vi "Autonomous_Load.vi"(0 "Number of Commands":i32, 5 "Subsystems":string[](array[string]), 7 "Commands":string[](array[string]), 9 "Inputs":string[][](array[string]), 11 "error in":errorcluster) -> (4 "Queue_Key":refnum<queue>, 6 "Autonomous_Queue":refnum<queue>, 15 "errror out":errorcluster)   [LabVIEW 2019]
uses:
  Queue_Key_Data.ctl
  Robot_Subsystems.ctl
  Subsystems/Drive/Drive_Cluster.ctl
  Subsystems/Drive/Drive_Control_States.ctl
  Subsystems/Drive/Drive_Orientation_States.ctl
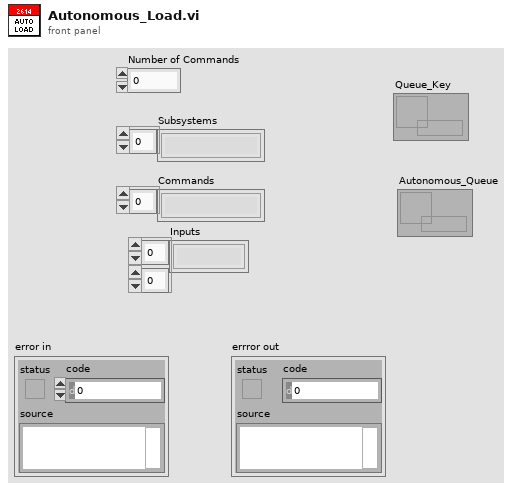
[diagram p1: front panel]
types:
  T1 = typedef "Robot_Subsystems.ctl" = cluster{"Drive_Cluster":T2}
  T2 = typedef "Drive_Cluster.ctl" = cluster{"Control_State":T3, "Vertical_Throttle":dbl, "Lateral_Throttle":dbl, "Rotational_Throttle":dbl, "Strafe_In_Deadband":bool, "Rotation_In_Deadband":bool, "Orientation_State":T4, "Parameters":dbl[], "Step":i32, "Auto_Notifier":refnum<notifier>}
  T3 = typedef "Drive_Control_States.ctl" = enum16{"Manual_Control", "Command_DriveDistanceAtAngle", ""}
  T4 = typedef "Drive_Orientation_States.ctl" = enum16{"Robot-Oriented", "Field-Oriented"}
  T5 = typedef "Queue_Key_Data.ctl" = cluster{"Operation Notifier":refnum<notifier>, "Subsystem":string, "Concurrent":bool}
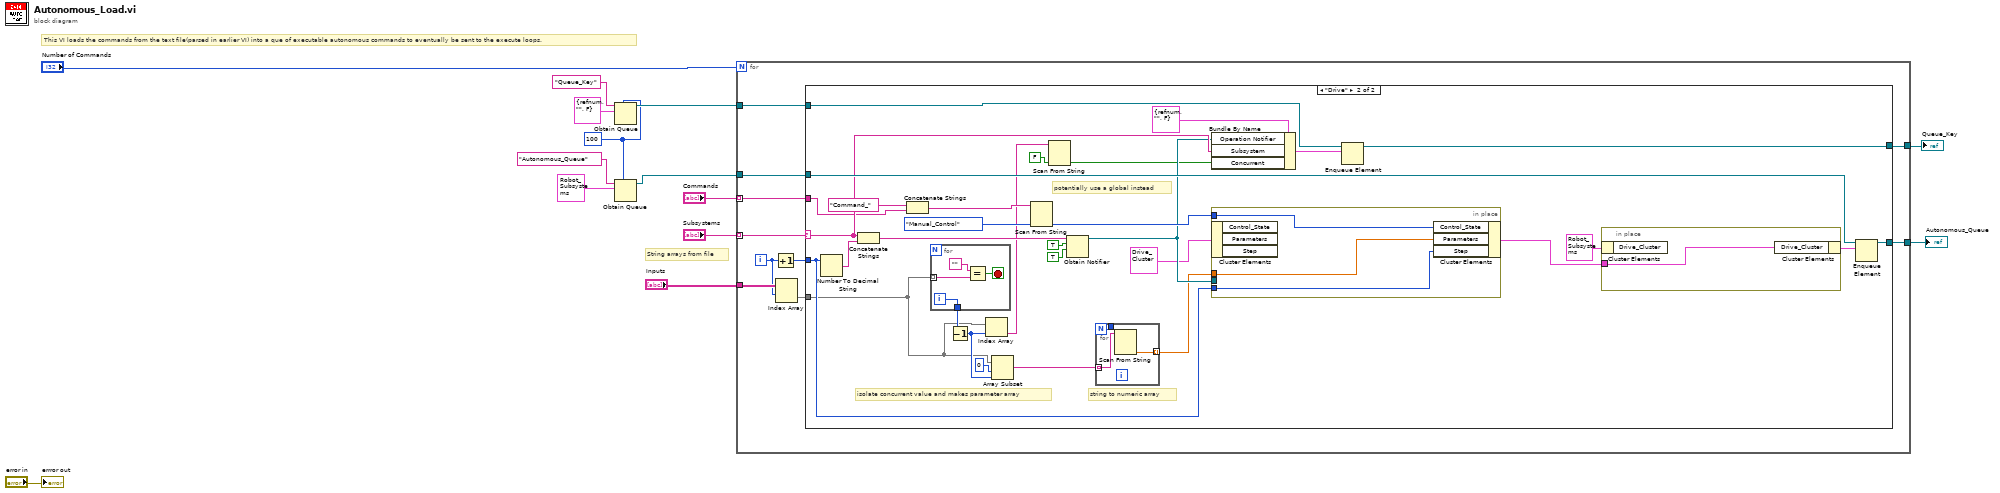
[diagram p0: block diagram]
diagram:
  w6 = 100 ("max queue size (-1, unlimited)")
  # "This VI loads the commands from the text file(parsed in earlier VI) into a que of executable autonomous commands to eventually be sent to the execute loops."
  # "String arrays from file"
  n1 = Obtain Queue(max queue size (-1, unlimited)=w6, name (unnamed)="Queue_Key", element data type=T5 {"Operation Notifier"=refnum, "Subsystem"="", "Concurrent"=FALSE} ("Queue Key Data")) -> (queue out=w12:refnum<queue>)  [unwired: 2 in, 2 out]
  n2 = Obtain Queue(max queue size (-1, unlimited)=w6, name (unnamed)="Autonomous_Queue", element data type=T1 {"Drive_Cluster"={"Control_State"=enum."Manual_Control", "Vertical_Throttle"=0.0, "Lateral_Throttle"=0.0, "Rotational_Throttle"=0.0, "Strafe_In_Deadband"=FALSE, "Rotation_In_Deadband"=FALSE, "Orientation_State"=enum."Robot-Oriented", "Parameters"=[], "Step"=0, "Auto_Notifier"=refnum}}) -> (queue out=w7:refnum<queue>)  [unwired: 2 in, 2 out]
  n3 = for {
    N: "Number of Commands" -> [_]
    tunnel: w12 -> [w24]
    tunnel: "Subsystems" -> [w23] mode=indexing
    tunnel: "Commands" -> [w22] mode=indexing
    tunnel: "Inputs" -> [w18]
    tunnel: [w21] -> w4
    tunnel: w7 -> [w20]
    tunnel: [w15] -> w1
    i -> [w16]
    n4 = Increment(x=w16) -> (x+1=w19:i32)
    n5 = Index Array(array=w18, index (row)=w16) -> (element=w17:string[])  [unwired: 1 in]
    n6 = case shown="\"Drive\"" w23 {
      selector: w23 -> [_ w44]
      tunnel: w24 -> [w25 w47]
      tunnel: w22 -> [_ w38]
      tunnel: [w26 w48] -> w15
      tunnel: [w25 w40] -> w21
      tunnel: w20 -> [w26 w51]
      tunnel: w19 -> [_ w52]
      tunnel: w17 -> [_ w30]
      frame "No Op", Default {
      }
      frame "Drive" {
        # "isolate concurrent value and makes parameter array"
        # "string to numeric array"
        # "potentially use a global instead"
        n7 = Number To Decimal String(number=w52) -> (decimal integer string=w55:string)  [unwired: 1 in]
        n8 = Concatenate Strings(w44, w55) -> (w54:string)
        n9 = Concatenate Strings("Command_" ("string"), w38) -> (w39:string)
        n10 = for {
          tunnel: w30 -> [w63] mode=indexing
          tunnel: [w62] -> w32
          i -> [w62]
          stop <- w61 stop-if-true
          n11 = Equal?(x="", y=w63) -> (x = y?=w61:bool)
        }
        n12 = Decrement(x=w32) -> (x-1=w33:i32)
        n13 = Index Array(array=w30, index=w33) -> (element=w29:string)
        n14 = Array Subset(array=w30, index=0, length=w33) -> (w28:string[])
        n15 = Scan From String(input string=w39, default 1=Drive_Control_States."Manual_Control" ("Control_State")) -> (output 1=w53:T3)  [unwired: 3 in, 3 out]
        n16 = Scan From String(input string=w29, default 1=FALSE) -> (output 1=w41:bool)  [unwired: 3 in, 3 out]
        n17 = Obtain Notifier(name (unnamed)=w54, notification data type=TRUE ("create if not found? (T)"), create if not found? (T)=TRUE) -> (notifier out=w43:refnum<notifier>)  [unwired: 1 in, 2 out]
        n18 = for {
          N -> [w58]
          tunnel: w28 -> [w60] mode=indexing
          tunnel: [w59] -> w27 mode=indexing
          tunnel: [w58] -> _
          n19 = Scan From String(input string=w60) -> (output 1=w59:dbl)  [unwired: 4 in, 3 out]
        }
        n20 = Bundle By Name(cluster=T5 {"Operation Notifier"=refnum, "Subsystem"="", "Concurrent"=FALSE} ("Queue Key Data"), "Operation Notifier"=w43, "Subsystem"=w44, "Concurrent"=w41) -> (w46:T5)
        n21 = in-place {
          in-place-border: w53 -> [w66]
          in-place-border: w43 -> [_]
          in-place-border: w52 -> [w68]
          in-place-border: w27 -> [w67]
          n22 = in-place-cluster #1(T2 {"Control_State"=enum."Manual_Control", "Vertical_Throttle"=0.0, "Lateral_Throttle"=0.0, "Rotational_Throttle"=0.0, "Strafe_In_Deadband"=FALSE, "Rotation_In_Deadband"=FALSE, "Orientation_State"=enum."Robot-Oriented", "Parameters"=[], "Step"=0, "Auto_Notifier"=refnum} ("Drive_Cluster")) -> ()  [unwired: 3 out]
          n23 = in-place-cluster #1("Control_State"=w66, "Parameters"=w67, "Step"=w68) -> (w50:T2)
        }
        n24 = Enqueue Element(queue=w47, element=w46) -> (queue out=w40:refnum<queue>)  [unwired: 2 in, 2 out]
        n25 = in-place {
          in-place-border: w50 -> [w65]
          n26 = in-place-cluster #2(T1 {"Drive_Cluster"={"Control_State"=enum."Manual_Control", "Vertical_Throttle"=0.0, "Lateral_Throttle"=0.0, "Rotational_Throttle"=0.0, "Strafe_In_Deadband"=FALSE, "Rotation_In_Deadband"=FALSE, "Orientation_State"=enum."Robot-Oriented", "Parameters"=[], "Step"=0, "Auto_Notifier"=refnum}}) -> ()  [unwired: 1 out]
          n27 = in-place-cluster #2("Drive_Cluster"=w65) -> (w49:T1)
        }
        n28 = Enqueue Element(queue=w51, element=w49) -> (queue out=w48:refnum<queue>)  [unwired: 2 in, 2 out]
      }
    }
  }
  "Queue_Key" <- w4
  "Autonomous_Queue" <- w1
  "errror out" <- "error in"
